vi "Write Symbol By Name.vi"(6 "Data":variant, 8 "Error In":errorcluster, 10 "Symbol Name":string, 11 "AMS Connection":T1) -> (0 "Error Out":errorcluster, 3 "Success":bool)   [LabVIEW 2019]
doc: "Write the symbol with <b>Symbol Name</b>. <b>Data</b> is a variant, accepting any LabVIEW data type although some may not be supported by the internal conversion.\n\nStrings are only supported with a fix length of 80 characters."
uses:
  <userlib>/PMA/High Level/PLC/PLC.lvlib
  <userlib>/PMA/TwinCAT ADS.lvlib
  <userlib>/PMA/Low Level/TypeDefs/AMS.ctl
  <userlib>/PMA/Low Level/TypeDefs/AMS Connection.ctl
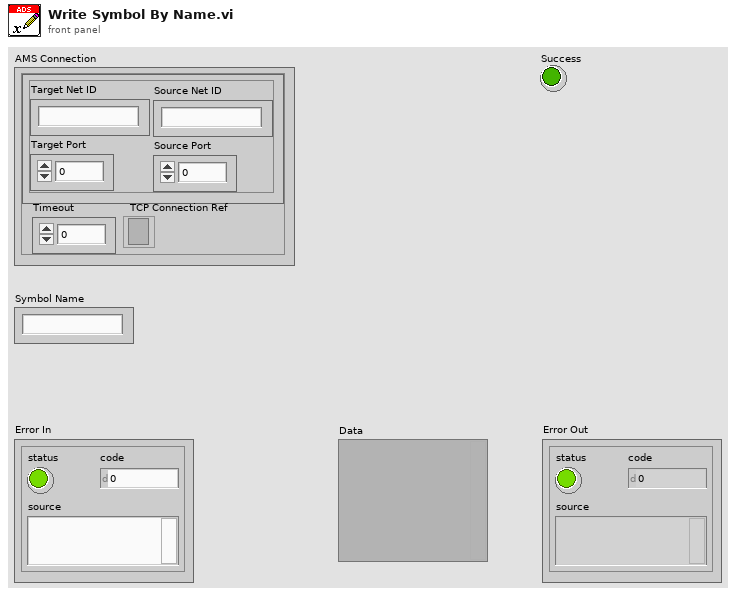
[diagram p1: front panel]
types:
  T1 = typedef "TwinCAT ADS.lvlib/AMS Connection.ctl" = cluster{"AMS":T2, "Timeout":i32, "TCP Connection Ref":refnum<k5>}
  T2 = typedef "TwinCAT ADS.lvlib/AMS.ctl" = cluster{"Target Net ID":string, "Target Port":u16, "Source Net ID":string, "Source Port":u16}
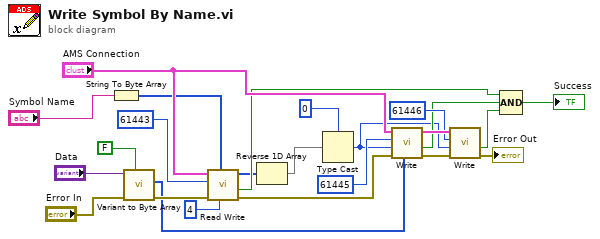
[diagram p0: block diagram]
diagram:
  n1 = String To Byte Array(string="Symbol Name") -> (unsigned byte array=w13:u8[])
  n2 = call <userlib>:"Variant to Byte Array.vi"("InStruct"=FALSE ("RISC"), "Error In"="Error In", "Variant"="Data") -> ("Error Out"=w22:errorcluster, "Byte Stream Out"=w21:u8[])  [unwired: 7 in]
  n3 = call <userlib>:"Read Write.vi"("Read Length"=u32 4, "Write Data"=w13, "Error In"=w22, "Index Group"=u32 61443, "AMS Connection In"="AMS Connection") -> ("Error Out"=w16:errorcluster, "Success"=w11:bool, "Read Data"=w4:u8[])  [unwired: 3 in, 1 out]
  n4 = Reverse 1D Array(array=w4) -> (reversed array=w5:u8[])
  n5 = Type Cast(type=u32 0, x=w5) -> (*(type *) &x=w7:u32)
  n6 = call <userlib>:"Write.vi"("Data"=w21, "Error In"=w16, "Offset"=w7, "Index Group"=u32 61445, "AMS Connection In"="AMS Connection") -> ("Error Out"=w15:errorcluster, "Success"=w9:bool, "AMS Connection Out"=w17:T1)  [unwired: 3 in, 1 out]
  n7 = call <userlib>:"Write.vi"("Error In"=w15, "Offset"=w7, "Index Group"=u32 61446, "AMS Connection In"=w17) -> ("Error Out"=→"Error Out":errorcluster, "Success"=w10:bool)  [unwired: 4 in, 2 out]
  n8 = Compound Arithmetic op=AND(w11, w9, w10) -> (→"Success":bool)
